vi "(SubVI) Stage Waveform Trigger_YCC.vi"(4 "Position Array (um)":dbl[](array[numeric]), 6 "milliseconds to wait":dbl, 7 "axis":u32) -> ()   [LabVIEW 2014]
uses:
  Main-Stage-PI/(Global) Current handle and LaserPower_YCC.vi
  MCL-dll-Labview 32-bit/Madlib.dll
panel:
  # "from 5 ms to 0.167 ms\n(20 Hz to 6000 Hz )"
  # "Max size = 6666 points"
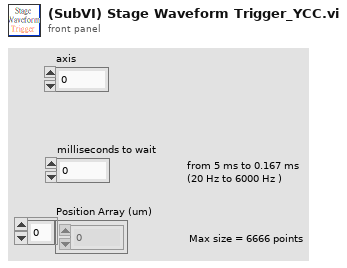
[diagram p1: front panel]
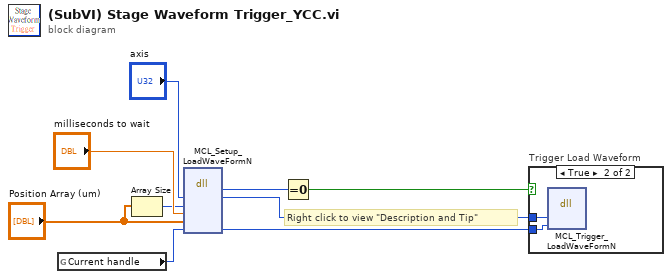
[diagram p0: block diagram]
diagram:
  # "Right click to view \"Description and Tip\""
  n1 = global read "(Global) Current handle and LaserPower_YCC.vi" "Current handle"() -> (w3:i32)
  n2 = Array Size(array="Position Array (um)") -> (size(s)=w1:i32)
  n3 = dll-call lib="C:/Users/hwlab/OneDrive - g.ntu.edu.tw/OT/YCC's OT-PI/Main-Stage-Based/SubVI-Stage-Based/MCL-dll-Labview 32-bit/MADLib.dll" fn="MCL_Setup_LoadWaveFormN" label="Setup WF Load"("axis"="axis", "DataPoints"=w1, "milliseconds"="milliseconds to wait", "waveform"="Position Array (um)", "handle"=w3) -> (w8:i32, "axis"=w7:u32, "handle"=w6:i32)  [unwired: 6 in, 2 out]
  n4 = Equal To 0?(x=w8) -> (x = 0?=w9:bool)
  n5 = case "Trigger Load Waveform" shown="True" w9 {
    tunnel: w7 -> [_ w11]
    tunnel: w6 -> [_ w10]
    frame False {
    }
    frame True {
      n6 = dll-call lib="C:/Users/hwlab/OneDrive - g.ntu.edu.tw/OT/YCC's OT-PI/Main-Stage-Based/SubVI-Stage-Based/MCL-dll-Labview 32-bit/MADLib.dll" fn="MCL_Trigger_LoadWaveFormN" ("Trigger Load Waveform")("axis"=w11, "handle"=w10) -> ()  [unwired: 6 in, 2 out]
    }
  }
